vi "NCO.vi"() -> ()   [LabVIEW 2013]
panel:
  out "M":dbl
  in  "N":i16=8
  in  "K":i32=1
  out "Waveform":dbl[](graph)
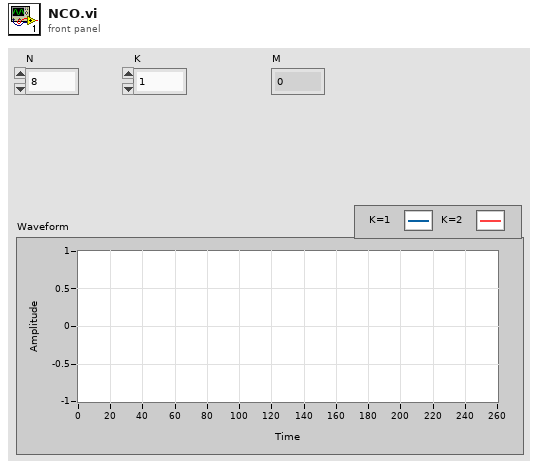
[diagram p1: front panel]
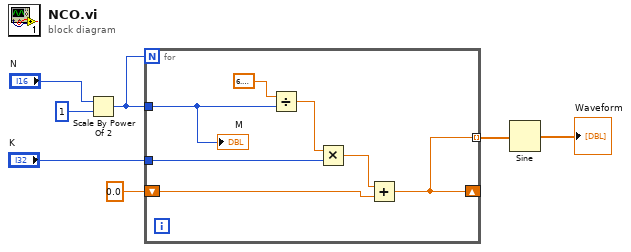
[diagram p0: block diagram]
diagram:
  n1 = Scale By Power Of 2(n="N", x=1) -> (x*2^n=w3:i32)
  n2 = for {
    N: w3 -> [_]
    tunnel: "K" -> [w12]
    shift-right: [w8] -> _
    shift-left: 0.0 -> [w10]
    tunnel: [w8] -> w2 mode=indexing
    tunnel: w3 -> [w9]
    n3 = Divide(x=6.283185307179586, y=w9) -> (x/y=w14:dbl)
    n4 = Multiply(x=w14, y=w12) -> (x*y=w11:dbl)
    n5 = Add(x=w11, y=w10) -> (x+y=w8:dbl)
    "M" <- w9
  }
  n6 = Sine(x=w2) -> (sin(x)=→"Waveform":dbl[])
